vi "CBL Set Baud Rate.vi"(5 "TimeOut":u32, 6 "BaudRate":u32, 7 "pInitConfig":T1, 9 "NodeAddr":u8, 10 "CANIndex":i32, 11 "DevIndex":i32) -> (2 "function return":i32, 3 "pInitConfig out":T1)   [LabVIEW 2010, in "CANBootloader.lvlib"]
doc: "int WINAPI CBL_SetBaudRate(int DevIndex,int CANIndex,unsigned char NodeAddr,PVCI_INIT_CONFIG_EX pInitConfig,unsigned int BaudRate,unsigned int TimeOut);"
uses:
  CANBootloader.lvlib
  CANBootloader/Ginkgo_Driver.dll
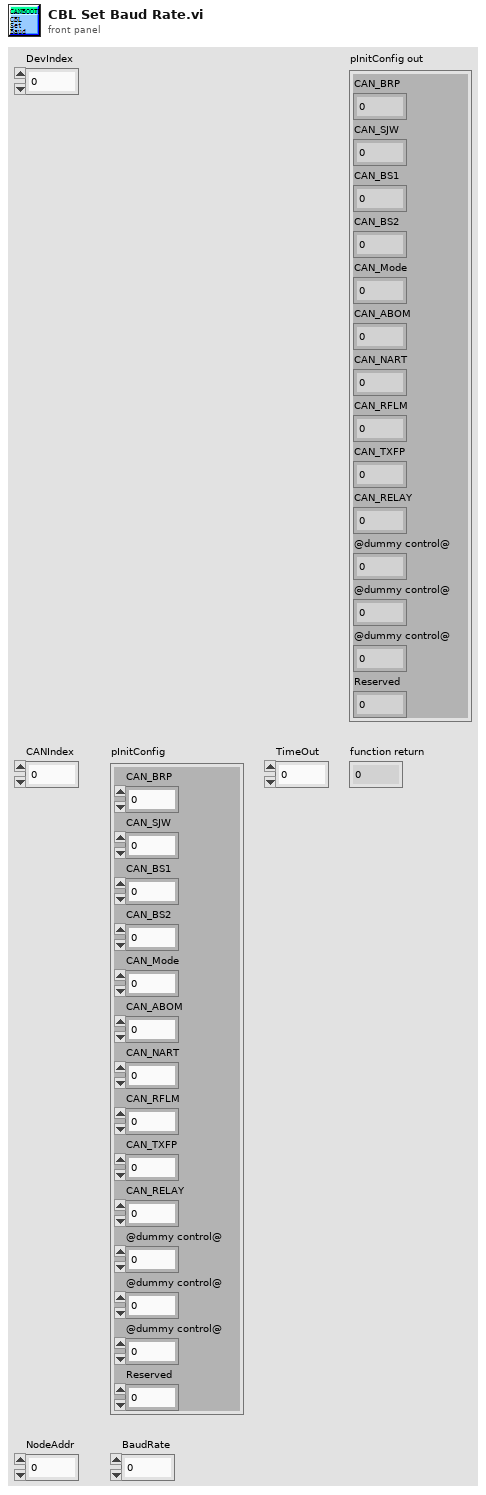
[diagram p1: front panel]
types:
  T1 = cluster{"CAN_BRP":u32, "CAN_SJW":u8, "CAN_BS1":u8, "CAN_BS2":u8, "CAN_Mode":u8, "CAN_ABOM":u8, "CAN_NART":u8, "CAN_RFLM":u8, "CAN_TXFP":u8, "CAN_RELAY":u8, "@dummy control@":i8, "@dummy control@":i8, "@dummy control@":i8, "Reserved":u32}
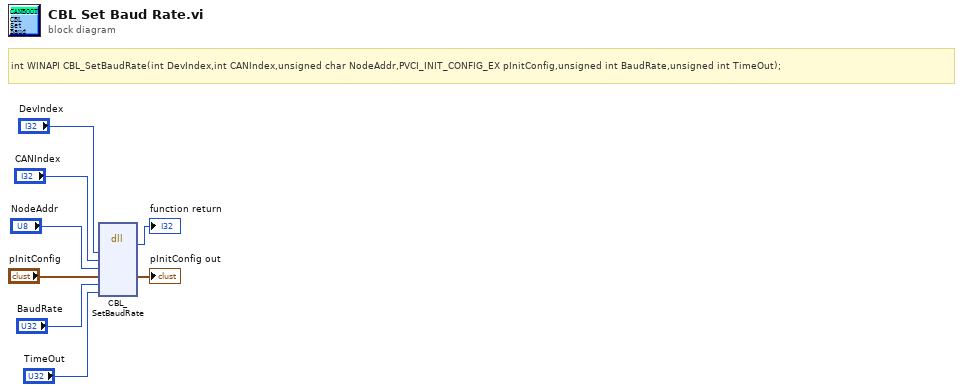
[diagram p0: block diagram]
diagram:
  # "int WINAPI CBL_SetBaudRate(int DevIndex,int CANIndex,unsigned char NodeAddr,PVCI_INIT_CONFIG_EX pInitConfig,unsigned int BaudRate,unsigned int TimeOut);"
  n1 = dll-call lib="E:/Project/vt_ginkgo/truck/Ginkgo Driver/vs2010/Ginkgo_USB-I2C&SPI&CAN_API_v2.0.3.3/lib/labview_32bit/CANBootloader/Ginkgo_Driver.*" fn="CBL_SetBaudRate"("DevIndex"="DevIndex", "CANIndex"="CANIndex", "NodeAddr"="NodeAddr", "pInitConfig"="pInitConfig", "BaudRate"="BaudRate", "TimeOut"="TimeOut") -> (→"function return":i32, "pInitConfig"=→"pInitConfig out":T1)  [unwired: 8 in, 2 out]
